vi "Assignment2_StudentList.vi"() -> ()   [LabVIEW 2024]
panel:
  out "No. of Students":i32
  out "Average Grade":dbl format="%#.2g"
  in  "Students":cluster{"Name":string[], "Grades":dbl[]}
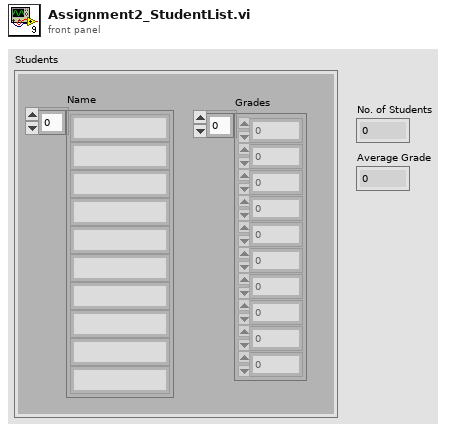
[diagram p1: front panel]
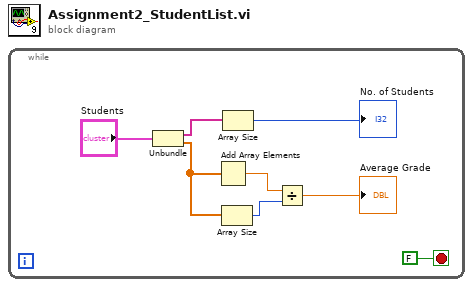
[diagram p0: block diagram]
diagram:
  n1 = while {
    stop <- FALSE stop-if-true
    n2 = Unbundle("Students") -> ("Name"=w7:string[], "Grades"=w2:dbl[])
    n3 = Add Array Elements(numeric array=w2) -> (sum=w4:dbl)
    n4 = Array Size(array=w2) -> (size(s)=w1:i32)
    n5 = Array Size(array=w7) -> (size(s)=→"No. of Students":i32)
    n6 = Divide(x=w4, y=w1) -> (x/y=→"Average Grade":dbl)
  }
